vi "LoadOrCreateATeststepIniCfg.vi"(8 "error in":errorcluster, 10 "Tree Refnum":refnum<vi>, 11 "Tbl Refnum in":refnum<vi>) -> (0 "error out":errorcluster, 1 "cfg file refnum out":refnum<file>, 2 "Tree Refnum out":refnum<vi>, 3 "Tbl Refnum out":refnum<vi>)   [LabVIEW 2010]
panel:
  out "All Tags":string[](array[string])
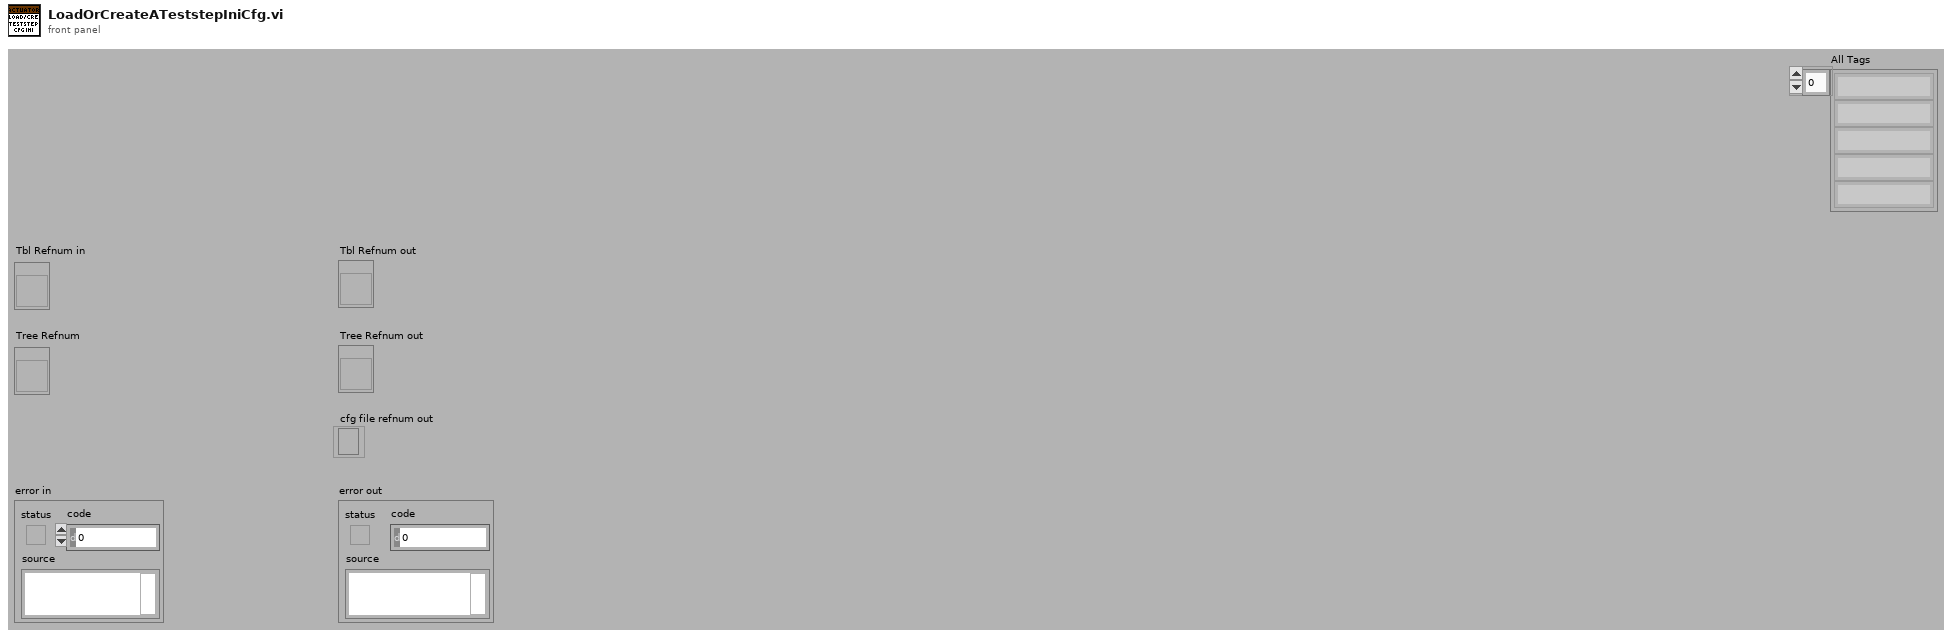
[diagram p1: front panel]
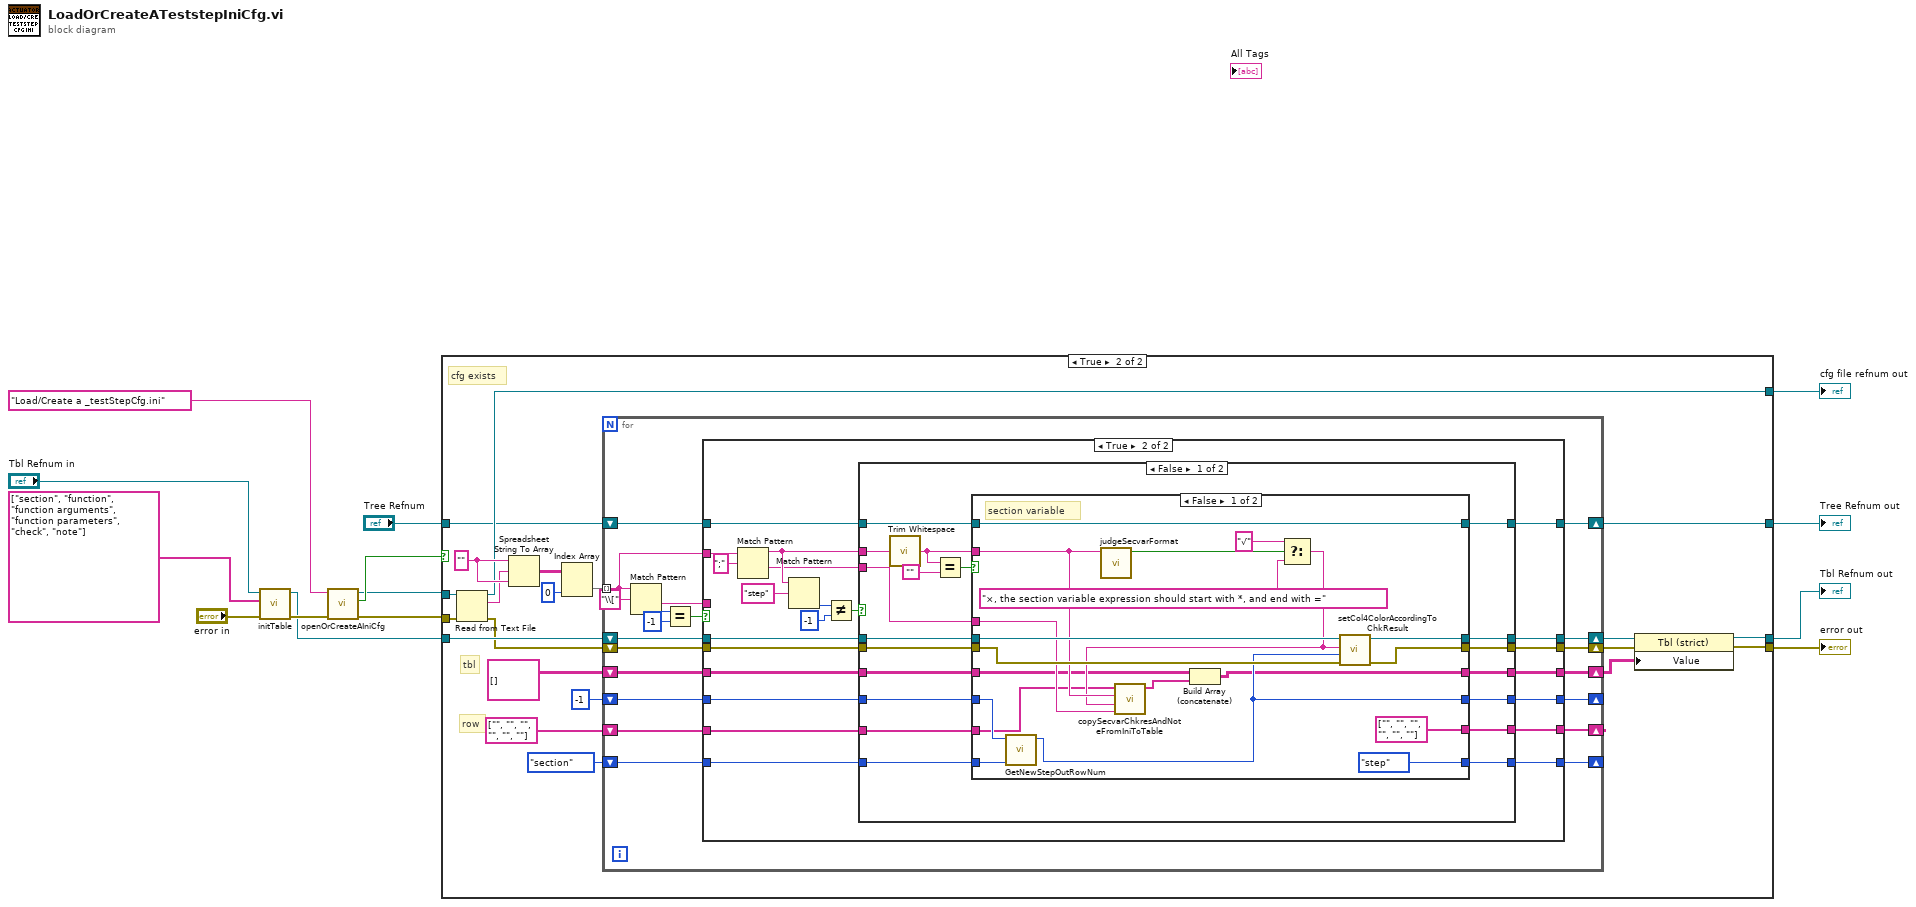
[diagram p0: block diagram]
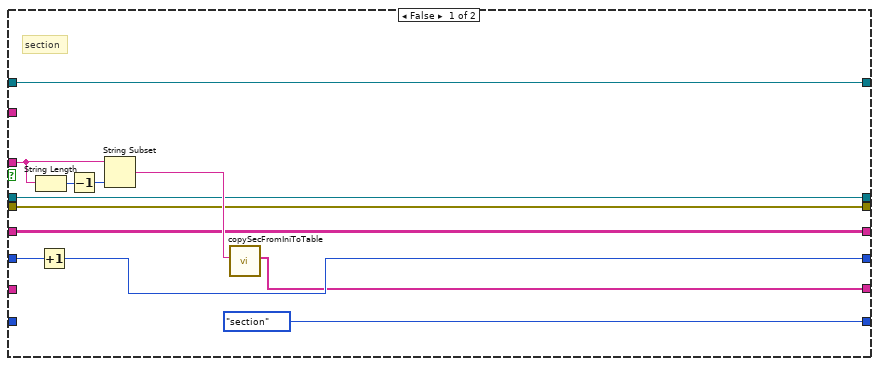
[diagram p3: hidden frame]
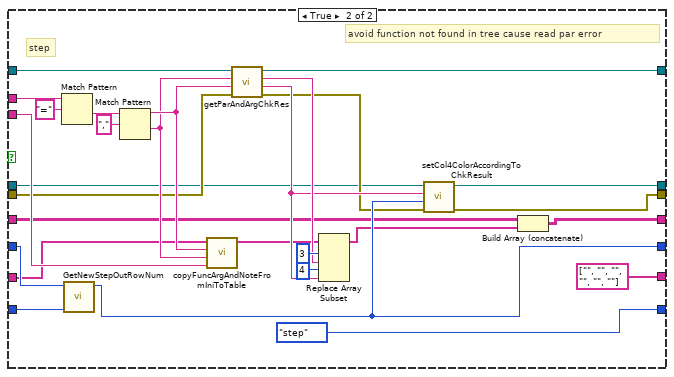
[diagram p5: hidden frame]
diagram:
  n1 = call "initTable.vi"("error in"="error in", "Column Header Strings[]"=string[] ["section", "function", "function arguments", "function parameters", "check", "note"] ("Row Header Strings[]"), "Tbl Refnum in"="Tbl Refnum in") -> ("error out"=w7:errorcluster, "Tbl Refnum out"=w2:refnum<vi>)  [unwired: 7 in]
  n2 = call "openOrCreateAIniCfg.vi"("error in"=w7, "prompt"="Load/Create a _testStepCfg.ini") -> ("error out"=w3:errorcluster, "exists"=w5:bool, "ini refnum out"=w4:refnum<file>)  [unwired: 7 in]
  n3 = case shown="True" w5 {
    tunnel: w4 -> [w18 w35]
    tunnel: w3 -> [w17 w34]
    tunnel: w2 -> [w16 w32]
    tunnel: [w18 w29] -> w14
    tunnel: [w17 w19] -> w13
    tunnel: [w16 w20] -> w12
    tunnel: "Tree Refnum" -> [w15 w27]
    tunnel: [w15 w26] -> w10
    frame False {
      # "create a new cfg"
    }
    frame True {
      w37 = ""
      # "row"
      # "tbl"
      # "cfg exists"
      n4 = Read from Text File(file (use dialog)=w35, error in=w34) -> (refnum out=w29:refnum<file>, text=w36:string, error out=w28:errorcluster)  [unwired: 2 in, 1 out]
      n5 = Spreadsheet String To Array(format string=w37, spreadsheet string=w36, array type (2D Dbl)=w37) -> (array=w38:string[][])  [unwired: 1 in]
      n6 = Index Array(array=w38, index (col)=0 ("disabled index (col)")) -> (element=w33:string[])  [unwired: 1 in]
      n7 = for {
        tunnel: w33 -> [w53] mode=indexing
        shift-right: [w51] -> _
        shift-left: -1 -> [w55]
        shift-right: [w50] -> _
        shift-left: enum16{"section", "step"}."section" -> [w49]
        shift-right: [w48] -> w22
        shift-left: w28 -> [w47]
        shift-right: [w46] -> w23
        shift-left: w32 -> [w52]
        shift-right: [w44] -> w26
        shift-left: w27 -> [w45]
        shift-right: [w42] -> w21
        shift-left: string[][] [] -> [w43]
        shift-right: [w41] -> _
        shift-left: string[] ["", "", "", "", "", ""] -> [w40]
        n8 = Match Pattern(string=w53, regular expression="\\[") -> (after substring=w54:string, offset past match=w58:i32)  [unwired: 1 in, 2 out]
        n9 = Equal?(x=w58, y=-1) -> (x = y?=w56:bool)
        n10 = case shown="True" w56 {
          tunnel: w55 -> [w68 w88]
          tunnel: [w62 w87] -> w51
          tunnel: w54 -> [w71 _]
          tunnel: w53 -> [_ w81]
          tunnel: w52 -> [w63 w89]
          tunnel: [enum16{"section", "step"}."section" w86] -> w50
          tunnel: w49 -> [_ w85]
          tunnel: w47 -> [w64 w84]
          tunnel: [w64 w83] -> w48
          tunnel: [w63 w82] -> w46
          tunnel: w45 -> [w66 w78]
          tunnel: [w66 w77] -> w44
          tunnel: w43 -> [w60 w75]
          tunnel: [w60 w74] -> w42
          tunnel: [w61 w72] -> w41
          tunnel: w40 -> [_ w73]
          frame False {
            # "section"
            n11 = String Length(string=w71) -> (length=w70:i32)
            n12 = Increment(x=w68) -> (x+1=w62:i32)
            n13 = Decrement(x=w70) -> (x-1=w69:i32)
            n14 = String Subset(string=w71, length (rest)=w69) -> (substring=w65:string)  [unwired: 1 in]
            n15 = call "copySecFromIniToTable.vi"("valInCol0"=w65) -> ("arrWithSec"=w61:string[])  [unwired: 10 in]
          }
          frame True {
            n16 = Match Pattern(string=w81, regular expression=";") -> (before substring=w79:string, after substring=w76:string)  [unwired: 1 in, 2 out]
            n17 = Match Pattern(string=w79, regular expression="step") -> (offset past match=w91:i32)  [unwired: 1 in, 3 out]
            n18 = Not Equal?(x=w91, y=-1) -> (x != y?=w93:bool)
            n19 = case shown="False" w93 {
              tunnel: w79 -> [w112 w166]
              tunnel: w89 -> [w110 w149]
              tunnel: w88 -> [w108 w162]
              tunnel: [w103 w152] -> w87
              tunnel: [w102 enum16{"section", "step"}."step"] -> w86
              tunnel: w85 -> [w107 w161]
              tunnel: w84 -> [w109 w156]
              tunnel: [w105 w148] -> w83
              tunnel: [w104 w147] -> w82
              tunnel: w78 -> [w101 w159]
              tunnel: [w100 w140] -> w77
              tunnel: w76 -> [w106 w160]
              tunnel: w75 -> [w97 w146]
              tunnel: [w96 w144] -> w74
              tunnel: w73 -> [w95 w143]
              tunnel: [w94 string[] ["", "", "", "", "", ""]] -> w72
              frame False {
                n20 = call <vilib>:"Trim Whitespace.vi"("string"=w112) -> ("trimmed string"=w98:string)  [unwired: 1 in]
                n21 = Equal?(x=w98, y="") -> (x = y?=w111:bool)
                n22 = case shown="False" w111 {
                  tunnel: w110 -> [w123 w139]
                  tunnel: w109 -> [w122 w138]
                  tunnel: w108 -> [w132 w137]
                  tunnel: w107 -> [w131 w136]
                  tunnel: w106 -> [w119 _]
                  tunnel: [w124 w138] -> w105
                  tunnel: [w125 w139] -> w104
                  tunnel: [w121 w137] -> w103
                  tunnel: [enum16{"section", "step"}."step" w136] -> w102
                  tunnel: [w130 w135] -> w100
                  tunnel: w101 -> [w130 w135]
                  tunnel: w98 -> [w120 _]
                  tunnel: w97 -> [w117 w134]
                  tunnel: [w116 w134] -> w96
                  tunnel: w95 -> [w115 w133]
                  tunnel: [string[] ["", "", "", "", "", ""] w133] -> w94
                  frame False {
                    # "section variable"
                    n23 = call "GetNewStepOutRowNum.vi"("lastStat"=w131, "lastRowNum"=w132) -> ("outRowNum"=w121:i32)  [unwired: 9 in]
                    n24 = call "judgeSecvarFormat.vi"("section variable"=w120) -> ("correct format?"=w128:bool)  [unwired: 10 in]
                    n25 = Select(t="√", s=w128, f="×, the section variable expression should start with *, and end with =" ("Value")) -> (s? t:f=w118:string)
                    n26 = call "copySecvarChkresAndNoteFromIniToTable.vi"("valInCol5"=w119, "valInCol4"=w118, "valInCol2"=w120, "arrayAtSameRow"=w115) -> ("arrWithSecvar&Chkres&Note"=w114:string[])  [unwired: 7 in]
                    n27 = Build Array (concatenate)(w117, w114) -> (w116:string[][])
                    n28 = call "setCol4ColorAccordingToChkResult.vi"("error in"=w122, "rowNum"=w121, "judgeRes"=w118, "Tbl Refnum in"=w123) -> ("error out"=w124:errorcluster, "Tbl Refnum Out"=w125:refnum<vi>)  [unwired: 6 in]
                  }
                  frame True {
                    # "blank"
                  }
                }
              }
              frame True {
                # "avoid function not found in tree cause read par error"
                # "step"
                n29 = Match Pattern(string=w166, regular expression="=") -> (after substring=w165:string)  [unwired: 1 in, 3 out]
                n30 = call "GetNewStepOutRowNum.vi"("lastStat"=w161, "lastRowNum"=w162) -> ("outRowNum"=w152:i32)  [unwired: 9 in]
                n31 = Match Pattern(string=w165, regular expression=",") -> (before substring=w158:string, after substring=w157:string)  [unwired: 1 in, 2 out]
                n32 = call "copyFuncArgAndNoteFromIniToTable.vi"("valInCol5"=w160, "valInCol2"=w157, "valInCol1"=w158, "arrayAtTheSameRow"=w143) -> ("arrWithFunc&Arg&Note"=w142:string[])  [unwired: 7 in]
                n33 = call "getParAndArgChkRes.vi"("error in"=w156, "func"=w158, "arg"=w157, "Tree Refnum in"=w159) -> ("error out"=w150:errorcluster, "Check result"=w151:string, "par"=w153:string, "Tree Refnum out"=w140:refnum<vi>)  [unwired: 4 in]
                n34 = Replace Array Subset(array=w142, new element #1=w153, index #1=3 ("index"), new element #2=w151, index #2=4 ("index")) -> (w145:string[])
                n35 = call "setCol4ColorAccordingToChkResult.vi"("error in"=w150, "rowNum"=w152, "judgeRes"=w151, "Tbl Refnum in"=w149) -> ("error out"=w148:errorcluster, "Tbl Refnum Out"=w147:refnum<vi>)  [unwired: 6 in]
                n36 = Build Array (concatenate)(w146, w145) -> (w144:string[][])
              }
            }
          }
        }
      }
      n37 = property class="Tbl (strict)"(reference=w23, error in=w22, "Value"=w21) -> (reference out=w20:refnum<vi>, error out=w19:errorcluster)
    }
  }
  "error out" <- w13
  "cfg file refnum out" <- w14
  "Tbl Refnum out" <- w12
  "Tree Refnum out" <- w10
